vi "Implement Publication Policy.vi"(8 "Publish Time":timestamp, 9 "New Value":variant, 10 "Previous Value":variant, 11 "MutexedPublishRequest":refnum<class "MutexedPublishRequest.lvclass">) -> (0 "error out":errorcluster, 2 "Value to Publish":variant)   [LabVIEW 2015, in "IMediator.lvlib" / "MutexedPublishRequest.lvclass"]
doc: "This method decides whether to or how to put the new data onto the bus. It allows the publish message to act as a mutex around varied types of publications. Publication policies like \"Increment Data\" allow the mediated data bus to perform FGV-like operations eliminating the risk of mediated data race conditions."
uses:
  MutexedPublishRequest.lvclass
  <vilib>/ErrorRing/Error Ring.xnode
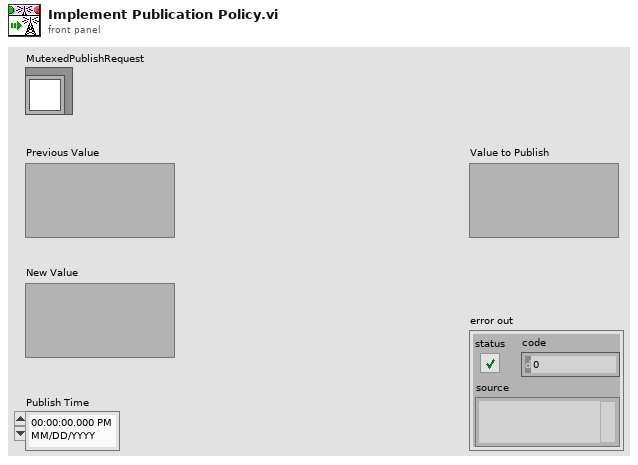
[diagram p1: front panel]
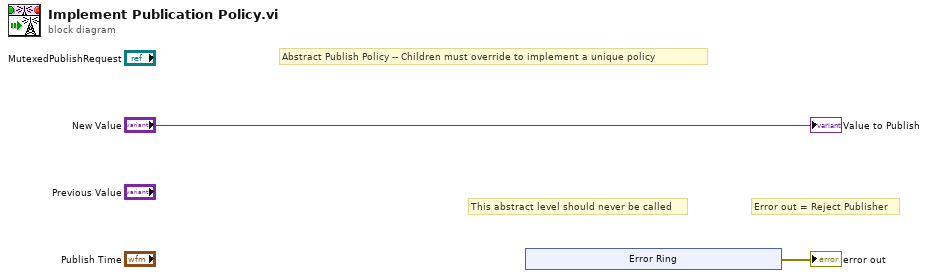
[diagram p0: block diagram]
diagram:
  # "This abstract level should never be called"
  # "Abstract Publish Policy -- Children must override to implement a unique policy"
  # "Error out = Reject Publisher"
  n1 = xnode "Error Ring"() -> ("error out"=→"error out":errorcluster)
  "Value to Publish" <- "New Value"
